vi "test_5160_stage2.vi"() -> ()   [LabVIEW 2013]
uses:
  <vilib>/measure/maspectr.llb/Power Spectrum and PSD Export Mode.ctl
  <vilib>/measure/maspectr.llb/FFT Power Spectrum and PSD for 1 Chan (CDB).vi
  <vilib>/measure/NI_MAPro.lvlib
  <vilib>/rvi/FXPMathLib/FxpInterpret/XNode/nifxpmath_Interpret.xnode
panel:
  out "size(s)":i32
  out "power spectrum after":cluster{"f0":dbl, "df":dbl, "magnitude":dbl[]}(graph)
  out "power spectrum bef":cluster{"f0":dbl, "df":dbl, "magnitude":dbl[]}(graph)
  out "Waveform Graph":i16[](graph)
  out "Iteration":i32
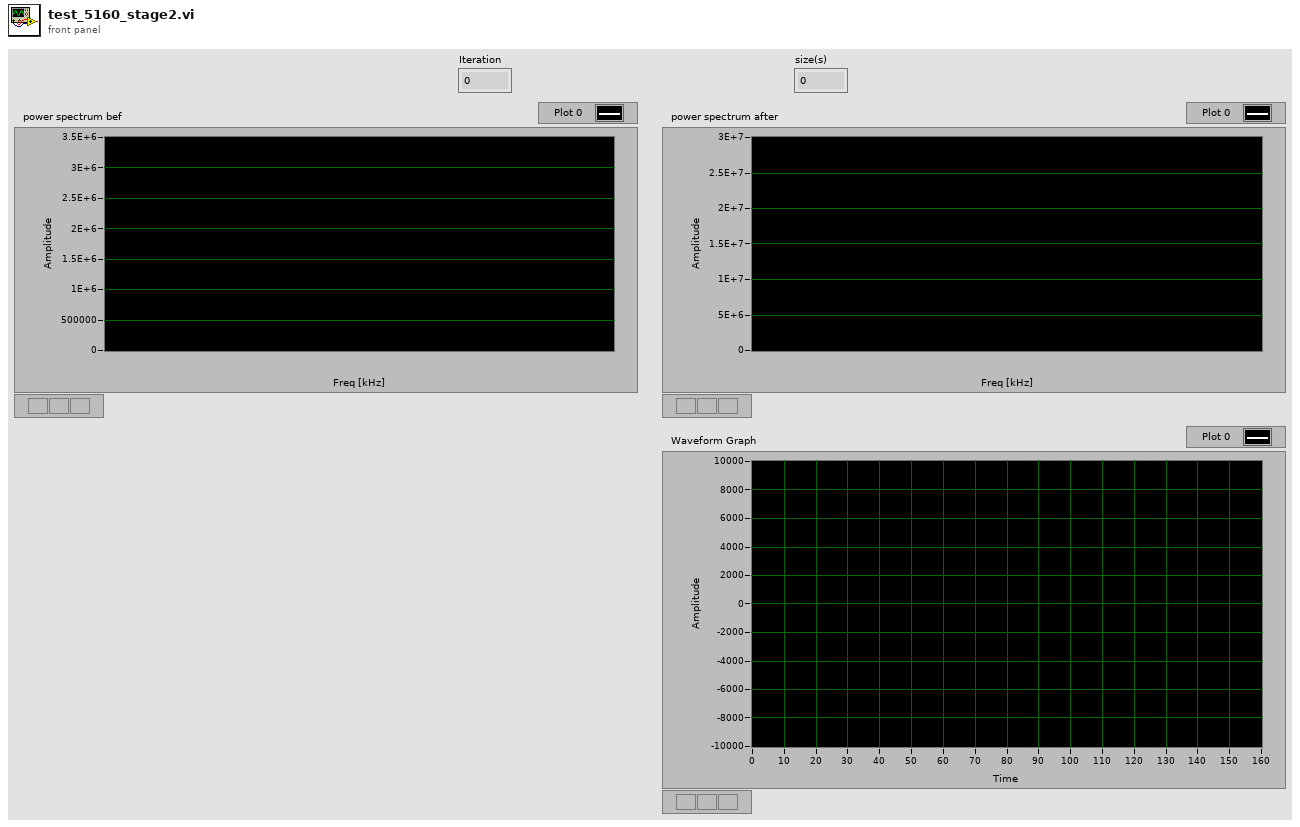
[diagram p1: front panel]
types:
  T1 = typedef "NI_MAPro.lvlib/Power Spectrum and PSD Export Mode.ctl" = u16
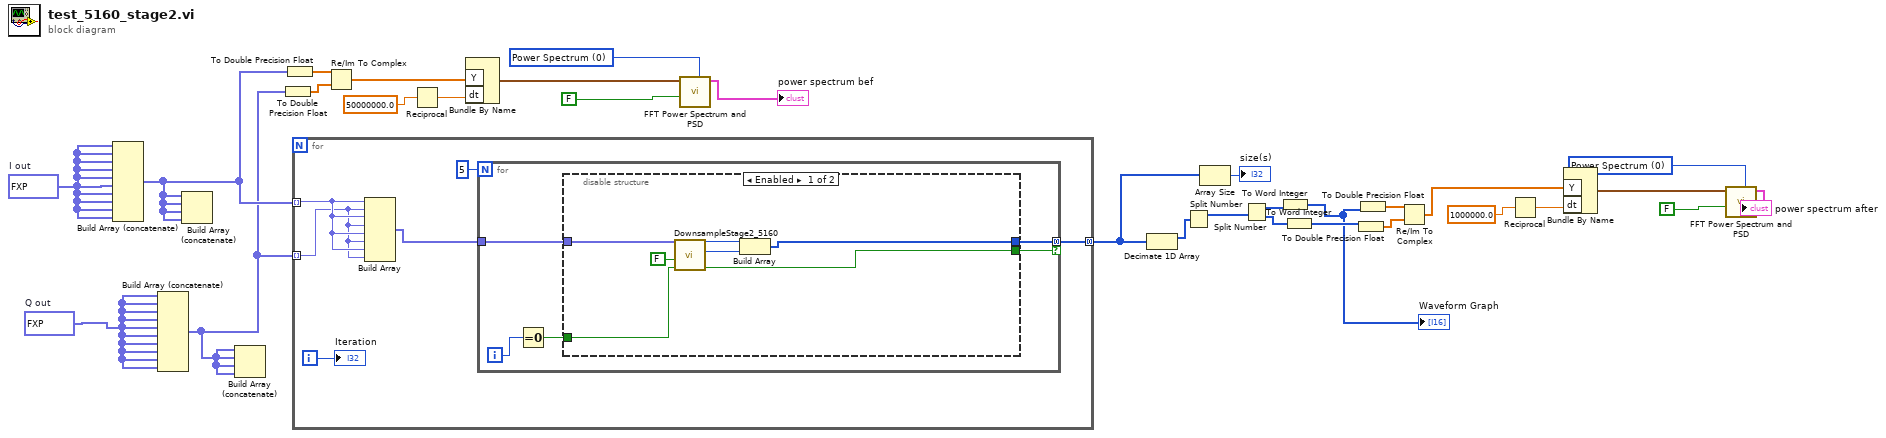
[diagram p0: block diagram]
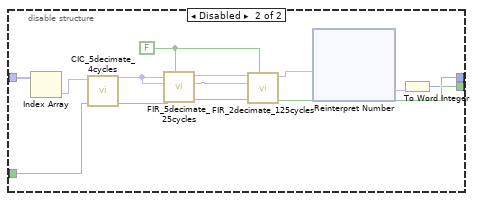
[diagram p2: hidden frame]
diagram:
  w14 = T1 0 items=["Power Spectrum", "Power Spectral Density"] ("export mode")
  w28 = T1 0 items=["Power Spectrum", "Power Spectral Density"] ("export mode")
  w29 = fxp<+/-,16,14>[] [0.0, -1.75, -30.0, 235.25, 2017.75, 3850.5, 3163.25, 910.0, 258.75, 2125.0, 3883.75, 3061.5, 812.5, 296.25, 2236.5, 3902.0, 2948.0, 711.75, 332.75, 2339.25, 3904.5, 2822.5, 608.0, 368.0, 2432.5, 3891.75, 2686.0, 502.25, 401.5, 2516.5, 3863.75, 2539.0, 394.0, 433.5, 2590.5, 3820.25, 2382.0, 284.5, 463.75, 2654.0, 3762.0, 2215.5, 174.0, 492.25, 2707.25, 3688.5, 2040.0, 62.5, 518.75, 2749.75, 3600.75, 1856.75, -49.0, 543.25, 2781.5, 3498.75, 1666.25, -160.5, 565.5, 2802.0, 3382.75, 1469.0, -271.25, 585.75, 2811.75, 3253.75, 1266.0, -381.0, 603.5, 2810.25, 3111.5, 1058.0, -489.25, 619.0, 2797.75, 2957.25, 845.75, -595.5, 631.75, 2774.25, 2791.0, 630.25, -699.5, 642.5, 2739.75, 2614.0, 412.25, -800.5, 650.25, 2694.25, 2426.75, 192.75, -898.5, 655.75, 2638.25, 2229.75, -28.0, -993.25, 658.25, 2572.0, 2024.0, -248.0, -1083.75, 658.5, 2495.25, 1810.25, -467.5, -1170.0, 656.25, 2409.0, 1589.5, -685.0, -1251.5, 651.25, 2313.0, 1362.5, -899.75, -1328.25, 643.5, 2208.0, 1129.75, -1110.75, -1399.75, 633.5, 2094.0, 892.75, -1317.75, -1465.75, 620.75, 1972.25, 652.25, -1519.25, -1526.0, 605.75, 1842.5, 409.0, -1715.0, -1580.0, 588.25, 1705.25, 164.25, -1904.0, -1628.25, 568.5, 1561.5, -81.0, -2085.25, -1669.5, 546.25, 1411.5, -326.0, -2258.5, -1704.5, 522.0, 1255.75, -569.5, -2422.75, -1732.5, 495.75, 1095.25, -811.25, -2577.5, -1754.0, 467.5, 930.5, -1049.5, -2722.0, -1768.5, 437.5, 762.0, -1283.75, -2855.75, -1775.75, 405.75, 590.5, -1512.75, -2978.25, -1776.25, 372.25, 416.5, -1736.0, -3089.0, -1769.75, 337.5, 241.0, -1952.25, -3187.5, -1756.25, 301.25, 64.75, -2160.75, -3273.5, -1735.75, 263.75, -112.0, -2361.0, -3346.5, -1708.5, 225.25, -288.5, -2551.75, -3406.5, -1674.25, 186.25, -463.5, -2732.5, -3453.0, -1633.75, 146.0, -636.75, -2902.25, -3485.5, -1586.5, 105.25, -807.5, -3060.75, -3504.75, -1533.25, 64.25, -975.25, -3207.0, -3509.75, -1473.75, 23.0, -1139.0, -3340.75, -3501.25, -1408.75, -18.5, -1298.25, -3461.25, -3478.75, -1338.0, -59.75, -1452.5, -3568.25, -3442.5, -1261.75, -101.0, -1600.75, -3661.0, -3392.75, -1180.75, -141.5, -1743.0, -3739.5, -3329.75, -1095.0, -181.75, -1878.25, -3803.0, -3253.25, -1005.0, -221.25, -2006.0, -3851.5, -3164.25, -911.0, -260.0, -2126.0, -3885.0, -3062.75, -813.5, -297.5, -2237.5, -3903.0, -2949.0, -712.75, -333.75, -2340.0, -3905.5, -2823.75, -609.0, -369.0, -2433.75, -3893.0, -2687.0, -503.0, -402.5, -2517.5, -3864.75, -2540.0, -395.0, -434.25, -2591.5, -3821.5, -2383.0, -285.5, -464.75, -2655.0, -3763.0, -2216.25, -174.75, -493.25, -2708.5, -3689.75, -2041.0, -63.5, -520.0, -2750.75, -3601.75, -1858.0, 48.0, -544.25, -2782.5, -3499.75, -1667.25, 159.5, -566.5, -2803.25, -3384.0, -1470.0, 270.25, -586.75, -2812.75, -3254.75, -1267.0, 380.0, -604.5, -2811.25, -3112.5, -1059.0, 488.25, -620.0, -2798.75, -2958.25, -846.75, 594.5, -632.75, -2775.25, -2792.25, -631.25, 698.5, -643.25, -2740.75, -2615.25, -413.25, 799.5, -651.25, -2695.25, -2427.75, -193.75, 897.5, -656.75, -2639.5, -2231.0, 26.75, 992.25, -659.5, -2572.75, -2025.0, 247.0, 1082.5, -659.5, -2496.25, -1811.25, 466.5, 1168.75, -657.0, -2410.0, -1590.5, 684.0, 1250.5, -652.0, -2314.0, -1363.25, 898.75, 1327.25, -644.5, -2209.0, -1130.75, 1110.0, 1398.75, -634.5, -2095.25, -893.75, 1316.75, 1464.75, -621.75, -1973.25, -653.25, 1518.25, 1525.0, -606.75, -1843.25, -410.25, 1714.0, 1579.0, -589.25, -1706.25, -165.5, 1903.0, 1627.0, -569.25, -1562.5, 80.0, 2084.25, 1668.5, -547.5, -1412.5, 325.0, 2257.5, 1703.5, -523.0, -1256.75, 568.75, 2421.75, 1731.75, -496.75, -1096.5, 810.25, 2576.5, 1753.0, -468.5, -931.5, 1048.5, 2720.75, 1767.5, -438.5, -763.0, 1282.75, 2854.75, 1775.0, -406.75, -591.5, 1512.0, 2977.25, 1775.25, -373.25, -417.5, 1735.0, 3087.75, 1768.75, -338.5, -242.25, 1951.25, 3186.5, 1755.25, -302.25, -65.75, 2159.75, 3272.5, 1734.75, -264.75, 111.0, 2360.0, 3345.5, 1707.5, -226.5, 287.25, 2550.75, 3405.5, 1673.5, -187.0, 462.5, 2731.25, 3451.75, 1632.75, -147.0, 635.75, 2901.25, 3484.5, 1585.5, -106.25, 806.75, 3059.75, 3503.75, 1532.25, -65.0, 974.25, 3206.0, 3508.75, 1473.0, -23.75, 1138.0, 3339.75, 3500.25, 1407.5, 17.5, 1297.25, 3460.25, 3477.75, 1336.75, 59.0, 1451.25, 3567.25, 3441.75, 1260.75, 99.75, 1599.75, 3660.0, 3391.75, 1179.75, 140.75, 1742.0, 3738.5, 3328.75, 1094.0, 180.75, 1877.0, 3802.0, 3252.5, 1004.0, 220.25, 2005.0, 3850.5, 3163.25, 910.0, 258.75, 2125.0, 3883.75, 3061.5, 812.5, 296.25, 2236.5, 3902.0, 2948.0, 711.75, 332.75, 2339.25, 3904.5, 2822.5, 608.0, 368.0, 2432.5, 3891.75, 2686.25, 502.25, 401.5, 2516.5, 3863.75, 2539.0, 394.0, 433.5, 2590.5, 3820.5, 2382.0, 284.5, 463.75, 2654.0, 3762.0, 2215.5, 174.0, 492.25, 2707.25, 3688.75, 2040.25, 62.5, 518.75, 2749.75, 3600.75, 1856.75, -49.0, 543.25, 2781.5, 3498.75, 1666.25, -160.5, 565.5, 2802.0, 3382.75, 1469.0, -271.25, 585.75, 2811.75, 3253.75, 1266.0, -381.0, 603.5, 2810.25, 3111.5, 1058.0, -489.25, 619.0, 2797.75, 2957.25, 846.0, -595.5, 631.75, 2774.25, 2791.0, 630.25, -699.25, 642.5, 2739.75, 2614.0, 412.25, -800.75, 650.25, 2694.25, 2426.75, 192.75, -898.5, 655.5, 2638.25, 2229.75, -27.75, -993.0, 658.25, 2572.0, 2024.25, -248.0, -1083.5, 658.5, 2495.25, 1810.25, -467.5, -1170.0, 656.25, 2409.0, 1589.5, -684.75, -1251.5, 651.25, 2313.0, 1362.5, -899.75, -1328.25, 643.5, 2208.0, 1129.75, -1110.75, -1399.75, 633.5, 2094.25, 892.75, -1317.75, -1465.75, 620.75, 1972.25, 652.25, -1519.25, -1526.0, 605.75, 1842.5, 409.25, -1715.0, -1580.0, 588.25, 1705.25, 164.5, -1904.0, -1628.25, 568.5, 1561.5, -80.75, -2085.25, -1669.5, 546.25, 1411.5, -326.0, -2258.5, -1704.5, 522.25, 1255.75, -569.5, -2422.75, -1732.5, 495.75, 1095.25, -811.25, -2577.5, -1754.0, 467.5, 930.5, -1049.5, -2722.0, -1768.5, 437.5, 762.0, -1283.75, -2855.75, -1775.75, 405.75, 590.5, -1512.75, -2978.0, -1776.25, 372.25, 416.5, -1736.0, -3089.0, -1769.75, 337.5, 241.0, -1952.25, -3187.5, -1756.25, 301.25, 64.75, -2160.75, -3273.5, -1735.75, 263.75, -112.0, -2361.0, -3346.5, -1708.5, 225.25, -288.5, -2551.5, -3406.5, -1674.25, 186.0, -463.5, -2732.25, -3453.0, -1633.75, 146.0, -636.75, -2902.25, -3485.5, -1586.5, 105.25, -807.5, -3060.75, -3504.75, -1533.25, 64.25, -975.25, -3207.0, -3509.75, -1473.75, 23.0, -1139.0, -3340.75, -3501.25, -1408.75, -18.5, -1298.25, -3461.25, -3478.75, -1338.0, -59.75, -1452.5, -3568.25, -3442.5, -1261.75, -101.0, -1600.75, -3661.0, -3392.75, -1180.75, -141.75, -1743.0, -3739.5, -3329.75, -1095.25, -181.75, -1878.25, -3803.0, -3253.5, -1005.0, -221.25, -2006.0, -3851.5, -3164.25, -911.0, -259.75, -2125.75, -3885.0, -3062.75, -813.5, -297.5, -2237.5, -3903.0, -2949.0, -712.75, -333.75, -2340.0, -3905.5, -2823.75, -609.0, -369.0, -2433.75, -3893.0, -2687.0, -503.0, -402.5, -2517.5, -3864.75, -2540.25, -395.0, -434.25, -2591.5, -3821.5, -2383.0, -285.5, -464.75, -2655.0, -3763.0, -2216.5, -174.75, -493.25, -2708.5, -3689.75, -2041.25, -63.5]  # Q out
  w30 = fxp<+/-,16,14>[] [0.0, -1.5, -80.5, 622.75, 1792.25, 558.0, -1561.75, -1516.5, 666.5, 1954.75, 573.0, -1499.75, -1313.25, 906.25, 2074.75, 585.25, -1432.0, -1104.75, 1142.5, 2186.5, 595.25, -1358.5, -892.0, 1374.25, 2289.75, 602.75, -1279.75, -675.75, 1600.75, 2384.0, 608.0, -1195.75, -456.75, 1820.75, 2468.75, 610.75, -1107.25, -235.75, 2033.25, 2543.75, 611.0, -1014.25, -14.25, 2238.25, 2608.75, 609.0, -917.5, 207.5, 2434.25, 2663.5, 604.75, -816.75, 428.5, 2620.75, 2707.75, 597.75, -713.0, 648.0, 2796.5, 2741.25, 588.5, -606.5, 864.75, 2961.5, 2764.0, 577.0, -497.5, 1078.0, 3115.0, 2775.75, 563.25, -386.5, 1287.0, 3256.0, 2776.5, 547.25, -274.0, 1491.0, 3384.0, 2766.5, 529.0, -160.5, 1689.0, 3498.75, 2745.5, 508.75, -46.25, 1880.5, 3599.75, 2713.5, 486.5, 68.25, 2064.5, 3686.5, 2670.75, 462.25, 182.25, 2240.25, 3758.5, 2617.75, 436.25, 295.75, 2407.25, 3816.0, 2554.25, 408.5, 407.75, 2564.75, 3858.25, 2480.5, 379.25, 518.25, 2712.0, 3885.25, 2397.25, 348.5, 627.0, 2849.0, 3897.25, 2304.5, 316.0, 733.0, 2974.25, 3893.5, 2202.5, 282.5, 836.25, 3088.0, 3874.5, 2092.0, 247.75, 936.0, 3189.5, 3840.25, 1973.0, 212.25, 1032.25, 3278.25, 3790.75, 1846.5, 176.0, 1124.5, 3354.5, 3726.25, 1712.5, 138.75, 1212.0, 3417.0, 3647.25, 1571.75, 101.25, 1295.0, 3466.25, 3553.75, 1424.75, 63.0, 1372.5, 3501.75, 3446.25, 1272.5, 24.75, 1445.0, 3523.5, 3325.0, 1114.75, -13.75, 1511.5, 3531.5, 3190.75, 952.75, -52.25, 1572.25, 3525.25, 3044.0, 787.0, -90.25, 1626.75, 3505.25, 2885.0, 618.25, -128.25, 1674.75, 3471.5, 2714.75, 447.0, -165.5, 1716.25, 3424.0, 2533.75, 274.0, -202.0, 1751.0, 3362.75, 2342.75, 99.75, -238.0, 1778.75, 3288.5, 2142.5, -74.75, -272.75, 1799.25, 3201.0, 1933.75, -248.75, -306.75, 1813.0, 3101.25, 1717.5, -422.0, -339.25, 1819.5, 2989.0, 1494.5, -593.75, -370.75, 1818.75, 2865.0, 1265.25, -763.0, -400.5, 1810.75, 2729.75, 1031.25, -929.25, -428.75, 1795.75, 2583.5, 793.25, -1091.75, -455.5, 1773.75, 2427.25, 552.0, -1250.0, -480.25, 1744.5, 2261.5, 308.75, -1403.25, -503.0, 1708.5, 2086.5, 64.0, -1551.25, -523.75, 1665.75, 1903.5, -180.75, -1692.75, -542.75, 1616.5, 1713.0, -425.0, -1827.75, -559.5, 1560.75, 1515.75, -667.5, -1955.75, -574.0, 1498.75, 1312.5, -907.25, -2075.75, -586.25, 1431.0, 1104.0, -1143.5, -2187.5, -596.25, 1357.5, 891.0, -1375.25, -2290.75, -603.75, 1278.75, 674.75, -1601.75, -2385.0, -609.0, 1194.75, 455.75, -1821.5, -2469.75, -611.75, 1106.25, 235.0, -2034.5, -2544.75, -612.0, 1013.25, 13.0, -2239.25, -2610.0, -610.0, 916.25, -208.75, -2435.25, -2664.5, -605.5, 815.75, -429.5, -2621.5, -2708.75, -598.75, 712.0, -648.75, -2797.5, -2742.25, -589.5, 605.5, -865.75, -2962.5, -2765.0, -578.0, 496.5, -1078.75, -3115.75, -2776.5, -564.25, 385.5, -1288.0, -3256.75, -2777.5, -548.25, 273.0, -1492.0, -3385.0, -2767.5, -530.0, 159.5, -1690.25, -3499.75, -2746.25, -509.5, 45.25, -1881.5, -3600.75, -2714.5, -487.5, -69.0, -2065.5, -3687.5, -2672.0, -463.25, -183.25, -2241.25, -3759.5, -2618.5, -437.25, -296.5, -2408.25, -3817.0, -2555.0, -409.5, -408.75, -2565.75, -3859.5, -2481.75, -380.0, -519.25, -2713.25, -3886.5, -2398.25, -349.0, -628.0, -2850.0, -3898.25, -2305.5, -317.0, -734.0, -2975.25, -3894.5, -2203.5, -283.5, -837.0, -3089.0, -3875.5, -2093.0, -249.0, -937.0, -3190.5, -3841.25, -1974.0, -213.25, -1033.0, -3279.5, -3791.75, -1847.5, -177.0, -1125.5, -3355.5, -3727.5, -1713.5, -139.75, -1213.0, -3418.25, -3648.25, -1572.75, -102.0, -1295.75, -3467.25, -3554.75, -1425.75, -64.0, -1373.5, -3502.75, -3447.25, -1273.25, -25.75, -1446.0, -3524.5, -3326.0, -1115.75, 12.75, -1512.75, -3532.5, -3191.75, -953.75, 51.25, -1573.25, -3526.25, -3044.75, -788.0, 89.25, -1627.75, -3506.25, -2886.0, -619.25, 127.0, -1675.75, -3472.5, -2715.75, -448.0, 164.25, -1717.25, -3425.0, -2534.75, -275.0, 201.0, -1752.0, -3363.75, -2343.75, -100.75, 237.0, -1779.75, -3289.5, -2143.5, 73.75, 272.0, -1800.5, -3202.0, -1934.75, 248.0, 305.75, -1814.0, -3102.25, -1718.5, 421.25, 338.5, -1820.5, -2990.0, -1495.5, 592.75, 369.75, -1819.75, -2865.75, -1266.25, 762.0, 399.5, -1811.75, -2730.75, -1032.5, 928.25, 427.75, -1796.75, -2584.5, -794.25, 1090.75, 454.5, -1774.75, -2428.25, -553.0, 1249.0, 479.25, -1745.5, -2262.25, -309.75, 1402.5, 502.0, -1709.5, -2087.5, -65.0, 1550.0, 523.0, -1666.75, -1904.5, 179.75, 1691.75, 541.75, -1617.5, -1714.0, 424.0, 1827.0, 558.5, -1561.75, -1516.75, 666.5, 1954.75, 573.0, -1499.75, -1313.25, 906.25, 2074.75, 585.25, -1432.0, -1105.0, 1142.5, 2186.5, 595.25, -1358.5, -892.0, 1374.25, 2289.75, 602.75, -1279.75, -675.75, 1600.75, 2384.0, 608.0, -1195.75, -456.75, 1820.75, 2468.75, 610.75, -1107.25, -236.0, 2033.25, 2543.75, 611.0, -1014.25, -14.25, 2238.25, 2608.75, 609.0, -917.5, 207.5, 2434.25, 2663.75, 604.75, -816.75, 428.5, 2620.5, 2707.75, 597.75, -713.0, 648.0, 2796.5, 2741.25, 588.5, -606.5, 864.75, 2961.5, 2764.0, 577.0, -497.5, 1078.0, 3114.75, 2775.75, 563.25, -386.5, 1287.0, 3256.0, 2776.5, 547.25, -274.0, 1490.75, 3383.75, 2766.5, 529.0, -160.5, 1689.0, 3498.75, 2745.5, 509.0, -46.25, 1880.5, 3599.75, 2713.5, 486.5, 68.25, 2064.5, 3686.5, 2670.75, 462.25, 182.0, 2240.25, 3758.5, 2617.75, 436.25, 295.5, 2407.25, 3816.0, 2554.25, 408.5, 407.75, 2564.75, 3858.25, 2480.5, 379.25, 518.25, 2712.25, 3885.25, 2397.25, 348.5, 627.0, 2849.0, 3897.25, 2304.5, 316.0, 733.0, 2974.25, 3893.5, 2202.5, 282.5, 836.25, 3088.0, 3874.5, 2092.0, 247.75, 936.0, 3189.5, 3840.25, 1973.25, 212.25, 1032.25, 3278.25, 3790.75, 1846.5, 176.0, 1124.25, 3354.5, 3726.25, 1712.5, 138.75, 1212.0, 3417.0, 3647.25, 1571.75, 101.25, 1295.0, 3466.25, 3553.75, 1424.75, 63.0, 1372.5, 3501.75, 3446.25, 1272.5, 24.75, 1445.0, 3523.5, 3325.0, 1114.75, -13.75, 1511.5, 3531.5, 3190.75, 952.75, -52.25, 1572.25, 3525.25, 3044.0, 787.0, -90.25, 1626.75, 3505.25, 2885.0, 618.25, -128.25, 1674.75, 3471.5, 2714.75, 447.0, -165.25, 1716.25, 3424.0, 2533.75, 274.0, -202.0, 1751.0, 3362.75, 2342.75, 99.75, -238.0, 1778.75, 3288.5, 2142.5, -74.75, -272.75, 1799.25, 3201.0, 1933.75, -248.75, -306.5, 1813.0, 3101.25, 1717.5, -422.0, -339.25, 1819.5, 2989.0, 1494.5, -593.75, -370.5, 1818.75, 2865.0, 1265.25, -763.0, -400.5, 1810.75, 2729.75, 1031.25, -929.25, -428.75, 1795.75, 2583.5, 793.25, -1091.75, -455.5, 1773.75, 2427.25, 552.0, -1250.0, -480.25, 1744.5, 2261.5, 308.75, -1403.25, -503.0, 1708.5, 2086.5, 64.0, -1551.0, -523.75, 1665.75, 1903.5, -180.75, -1692.75, -542.75, 1616.5, 1713.0, -425.0, -1827.75, -559.5, 1560.75, 1515.75, -667.5, -1955.75, -574.0, 1498.75, 1312.5, -907.25, -2075.75, -586.25, 1431.0, 1104.0, -1143.5, -2187.5, -596.25, 1357.5, 891.0, -1375.25, -2290.75, -603.75, 1278.75, 674.75, -1601.75, -2385.0, -609.0, 1195.0, 455.75, -1821.5, -2469.75, -611.75, 1106.25, 235.0, -2034.25, -2544.75, -612.0, 1013.25, 13.25, -2239.25, -2610.0, -610.0, 916.25, -208.75]  # I out
  n1 = Build Array (concatenate)(w30, w30, w30, w30, w30, w30, w30, w30, w30, w30) -> (w3:fxp<+/-,16,14>[])
  n2 = Build Array (concatenate)(w29, w29, w29, w29, w29, w29, w29, w29, w29, w29) -> (w2:fxp<+/-,16,14>[])
  n3 = Build Array (concatenate)(w3, w3, w3, w3) -> ()  [unwired: 1 out]
  n4 = Build Array (concatenate)(w2, w2, w2, w2) -> ()  [unwired: 1 out]
  n5 = To Double Precision Float(number=w2) -> (double precision float=w21:dbl[])
  n6 = To Double Precision Float(number=w3) -> (double precision float=w22:dbl[])
  n7 = for {
    tunnel: w3 -> [w36] mode=indexing
    tunnel: w2 -> [w35] mode=indexing
    tunnel: [w31] -> w1 mode=concatenating
    i -> [w34]
    n8 = Build Array(w36, w35, w36, w35, w36, w35, w36, w35) -> (w33:fxp<+/-,16,14>[])
    n9 = for {
      N: 5 -> [_]
      tunnel: w33 -> [w41]
      tunnel: [w38] -> w31 mode=concatenating if=w39
      i -> [w40]
      n10 = Equal To 0?(x=w40) -> (x = 0?=w37:bool)
      n11 = disable-structure shown="Enabled" {
        disable-tunnel: w41 -> [w48 w55]
        disable-tunnel: [w46 w53] -> w39
        disable-tunnel: [w42 w50] -> w38
        disable-tunnel: w37 -> [w45 w49]
        frame Enabled {
          n12 = call "DownsampleStage2_5160.vi"("valid in"=w45, "reset"=FALSE, "Element"=w48) -> ("valid out"=w46:bool, "Element 2"=w43:u64, "Element 1"=w44:u64)  [unwired: 6 in]
          n13 = Build Array(w44, w43) -> (w42:u64[])
        }
        frame Disabled {
          w57 = FALSE ("reset")
          n14 = Index Array(array=w55) -> (element=w54:fxp<+/-,16,14>)  [unwired: 1 in]
          n15 = call "CIC_5decimate_4cycles.vi"("valid in"=w49, "Data in"=w54) -> ("valid out"=w60:bool, "Data out"=w61:fxp<+/-,16,14>)  [unwired: 7 in, 1 out]
          n16 = call "FIR_5decimate_25cycles.vi"("reset"=w57, "valid in"=w60, "Q in"=w61, "I in"=w61) -> ("valid out"=w56:bool, "Q out"=w58:fxp<+/-,16,14>, "I out"=w59:fxp<+/-,16,14>)  [unwired: 4 in, 1 out]
          n17 = call "FIR_2decimate_125cycles.vi"("reset"=w57, "valid in"=w56, "Q in"=w58, "I in"=w59) -> ("valid out"=w53:bool, "I out"=w51:fxp<+/-,16,14>)  [unwired: 4 in, 2 out]
          n18 = xnode "Reinterpret Number"("x"=w51) -> ("y"=w52:fxp<+/-,16,16>)
          n19 = To Word Integer(number=w52) -> (16bit integer=w50:i16)
        }
      }
    }
    "Iteration" <- w34
  }
  n20 = Re/Im To Complex(1:w21, 2:w22) -> (0:w20:cdb[])
  n21 = Reciprocal(x=50000000.0 ("dt")) -> (1/x=w24:dbl)
  n22 = Bundle By Name("Y"=w20, "dt"=w24) -> (w27:waveform(cdb))  [unwired: 1 in]
  n23 = call-poly <vilib>:"FFT Power Spectrum and PSD.vi"("export mode"=w28, "dB On (F)"=FALSE, "time signal"=w27) -> ("Power Spectrum / PSD"=→"power spectrum bef":cluster{"f0":dbl, "df":dbl, "magnitude":dbl[]})  [unwired: 5 in, 3 out]
  n24 = Decimate 1D Array(w1) -> (w5:u64[])  [unwired: 1 out]
  n25 = Split Number(x=w5) -> (hi(x)=w10:u32[])  [unwired: 1 out]
  n26 = Array Size(array=w1) -> (size(s)=→"size(s)":i32)
  n27 = Split Number(x=w10) -> (hi(x)=w9:u16[], lo(x)=w8:u16[])
  n28 = To Word Integer(number=w9) -> (16bit integer=w6:i16[])
  "Waveform Graph" <- w6
  n29 = To Word Integer(number=w8) -> (16bit integer=w7:i16[])
  n30 = To Double Precision Float(number=w7) -> (double precision float=w13:dbl[])
  n31 = To Double Precision Float(number=w6) -> (double precision float=w12:dbl[])
  n32 = Re/Im To Complex(1:w13, 2:w12) -> (0:w11:cdb[])
  n33 = Reciprocal(x=1000000.0 ("dt")) -> (1/x=w18:dbl)
  n34 = Bundle By Name("Y"=w11, "dt"=w18) -> (w15:waveform(cdb))  [unwired: 1 in]
  n35 = call-poly <vilib>:"FFT Power Spectrum and PSD.vi"("export mode"=w14, "dB On (F)"=FALSE, "time signal"=w15) -> ("Power Spectrum / PSD"=→"power spectrum after":cluster{"f0":dbl, "df":dbl, "magnitude":dbl[]})  [unwired: 5 in, 3 out]
